vi "Pressure Read Loop.vi"(0 "Pressure Graph Array Ref":refnum<vi>[](array[refnum]), 1 "Pressure (mTorr) Array Ref":refnum<vi>[](array[refnum]), 2 "Number of Reactors":i32=5, 3 "Logging Data Array Ref":refnum<vi>[](array[refnum]), 4 "Pressure Scale Array":refnum<vi>[](array[refnum]), 5 "Pressure Voltage\nCorrect Array":refnum<vi>[](array[refnum]), 9 "Queue Array Ref":refnum<vi>[](array[refnum]), 11 "Debug Mode":refnum<vi>, 12 "Reactor Selector":T1(ring), 13 "Stop Program":refnum<vi>, 15 "Current Cycle Reactor X":refnum<vi>[](array[refnum]), 17 "Start Time Reactor X":refnum<vi>[](array[refnum]), 19 "GUID X":refnum<vi>[](array[refnum])) -> ()   [LabVIEW 2021]
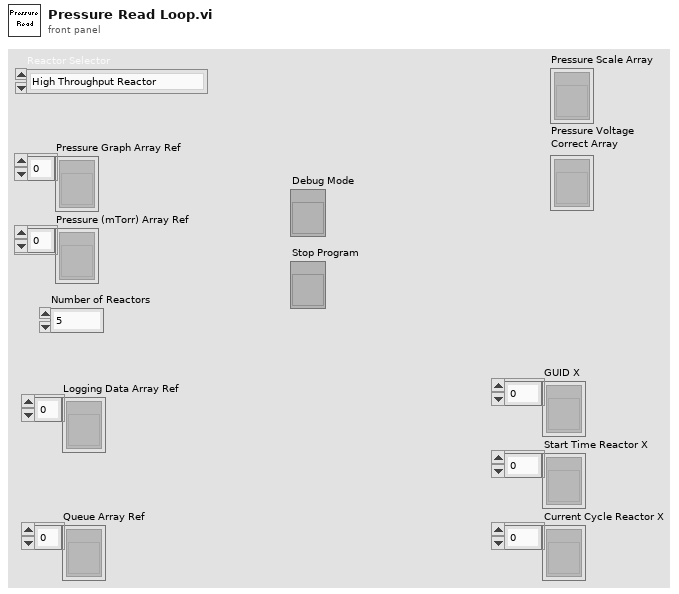
[diagram p1: front panel]
types:
  T1 = enum16{"High Throughput Reactor", "In Situ Reactor", "MLD Reactor"}
  T2 = cluster{"type":string, "meta":string, "payload":string}
  T3 = cluster{"TimeElapsed":string, "CurrentCycle":string, "Pressure":string, "GUID":string}
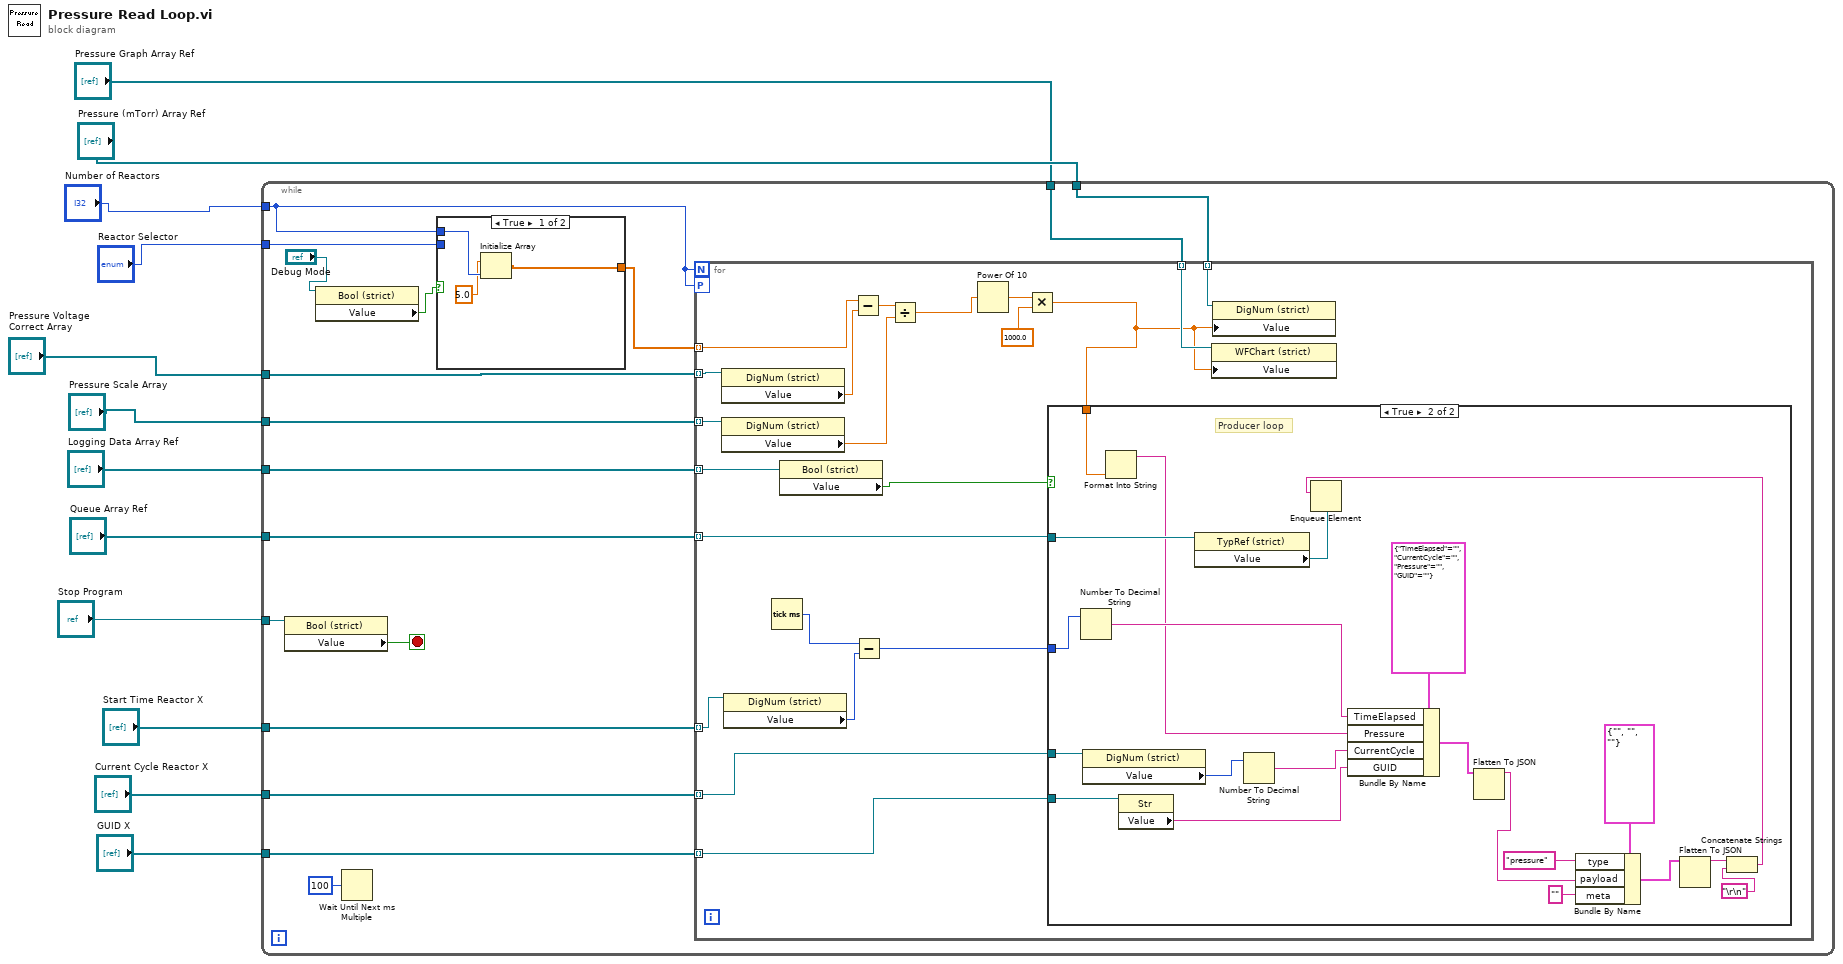
[diagram p0: block diagram]
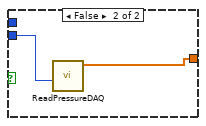
[diagram p2: hidden frame]
diagram:
  n1 = while {
    tunnel: "Pressure (mTorr) Array Ref" -> [w28]
    tunnel: "Pressure Graph Array Ref" -> [w27]
    tunnel: "Logging Data Array Ref" -> [w26]
    tunnel: "Queue Array Ref" -> [w25]
    tunnel: "Number of Reactors" -> [w24]
    tunnel: "Stop Program" -> [w21]
    tunnel: "Pressure Voltage\nCorrect Array" -> [w20]
    tunnel: "Pressure Scale Array" -> [w19]
    tunnel: "Reactor Selector" -> [w18]
    tunnel: "GUID X" -> [w17]
    tunnel: "Current Cycle Reactor X" -> [w16]
    tunnel: "Start Time Reactor X" -> [w15]
    stop <- w22 stop-if-true
    n2 = property class="Bool (strict)"(reference=w21) -> ("Value"=w22:bool)  [unwired: 1 in, 2 out]
    n3 = property class="Bool (strict)"(reference="Debug Mode") -> ("Value"=w14:bool)  [unwired: 1 in, 2 out]
    n4 = Wait Until Next ms Multiple(millisecond multiple=u32 100) -> ()  [unwired: 1 out]
    n5 = case shown="True" w14 {
      tunnel: [w32 w34] -> w13
      tunnel: w24 -> [w31 _]
      tunnel: w18 -> [_ w33]
      frame True {
        n6 = Initialize Array(5.0 ("element"), w31) -> (w32:dbl[])
      }
      frame False {
        n7 = call "ReadPressureDAQ.vi"("Reactor Selector"=w33) -> ("Array"=w34:dbl[])  [unwired: 10 in]
      }
    }
    n8 = for {
      N: w24 -> [_]
      workers-P: w24 -> [_]
      tunnel: w28 -> [w55] mode=indexing
      tunnel: w27 -> [w54] mode=indexing
      tunnel: w26 -> [w53] mode=indexing
      tunnel: w25 -> [w51] mode=indexing
      tunnel: w13 -> [w37] mode=indexing
      tunnel: w20 -> [w49] mode=indexing
      tunnel: w19 -> [w47] mode=indexing
      tunnel: w17 -> [w41] mode=indexing
      tunnel: w16 -> [w40] mode=indexing
      tunnel: w15 -> [w36] mode=indexing
      n9 = property class="DigNum (strict)"(reference=w49) -> ("Value"=w48:dbl)  [unwired: 1 in, 2 out]
      n10 = property class="DigNum (strict)"(reference=w47) -> ("Value"=w43:dbl)  [unwired: 1 in, 2 out]
      n11 = property class="DigNum (strict)"(reference=w36) -> ("Value"=w35:i32)  [unwired: 1 in, 2 out]
      n12 = Tick Count (ms)() -> (millisecond timer value=w39:u32)
      n13 = property class="Bool (strict)"(reference=w53) -> ("Value"=w52:bool)  [unwired: 1 in, 2 out]
      n14 = Subtract(x=w37, y=w48) -> (x-y=w44:dbl)
      n15 = Subtract(x=w39, y=w35) -> (x-y=w38:u32)
      n16 = Divide(x=w44, y=w43) -> (x/y=w42:dbl)
      n17 = Power Of 10(x=w42) -> (10^x=w50:dbl)
      n18 = Multiply(x=w50, y=1000.0) -> (x*y=w46:dbl)
      n19 = case shown="True" w52 {
        tunnel: w46 -> [_ w74]
        tunnel: w51 -> [_ w76]
        tunnel: w41 -> [_ w72]
        tunnel: w40 -> [_ w70]
        tunnel: w38 -> [_ w68]
        frame False {
        }
        frame True {
          # "Producer loop"
          n20 = Number To Decimal String(number=w68) -> (decimal integer string=w65:string)  [unwired: 1 in]
          n21 = property class="DigNum (strict)"(reference=w70) -> ("Value"=w69:i32)  [unwired: 1 in, 2 out]
          n22 = Format Into String(w74) -> (resulting string=w56:string)  [unwired: 3 in, 1 out]
          n23 = property class="Str"(reference=w72) -> ("Value"=w71:string)  [unwired: 1 in, 2 out]
          n24 = property class="TypRef (strict)"(reference=w76) -> ("Value"=w75:refnum<queue>)  [unwired: 1 in, 2 out]
          n25 = Number To Decimal String(number=w69) -> (decimal integer string=w64:string)  [unwired: 1 in]
          n26 = Bundle By Name(cluster=T3 {"TimeElapsed"="", "CurrentCycle"="", "Pressure"="", "GUID"=""} ("input cluster"), "TimeElapsed"=w65, "Pressure"=w56, "CurrentCycle"=w64, "GUID"=w71) -> (w60:T3)
          n27 = Flatten To JSON(anything=w60) -> (JSON string=w57:string)  [unwired: 2 in, 1 out]
          n28 = Bundle By Name(cluster=T2 {"type"="", "meta"="", "payload"=""} ("input cluster"), "type"="pressure", "payload"=w57, "meta"="") -> (w63:T2)
          n29 = Flatten To JSON(anything=w63) -> (JSON string=w61:string)  [unwired: 2 in, 1 out]
          n30 = Concatenate Strings(w61, "\r\n") -> (w58:string)
          n31 = Enqueue Element(queue=w75, element=w58) -> ()  [unwired: 2 in, 3 out]
        }
      }
      n32 = property class="WFChart (strict)"(reference=w54, "Value"=w46) -> ()  [unwired: 1 in, 2 out]
      n33 = property class="DigNum (strict)"(reference=w55, "Value"=w46) -> ()  [unwired: 1 in, 2 out]
    }
  }
